vi "Main.vi"() -> ()   [LabVIEW 2017]
doc: "32 channel relay control"
uses:
  Event clusterr.ctl
  EventMsg.ctl
  Sequence cluster.ctl
  SequenceMsg.ctl
  LowLevel cluster.ctl
  LowLevelMsg.ctl
  <vilib>/Utility/file.llb/Read Delimited Spreadsheet (I64).vi
panel:
  out "Current command to Arduino":string
  in  "clear error":bool
  in  "Arduino VISA resource name":refnum<visa-resource-name>
  in  "Exit":bool
  out "ERROR OUT":errorcluster
  in  "Frequency":dbl
  in  "RUN/STOP Signal":bool
  in  "RESET":bool
  out "StopLED":bool
  out "Current step":dbl=-1.0
  in  "Load File":bool
  in  "Path":path
  in  "Next":bool
  in  "Play":bool
  in  "Back":bool
  # "32-channel Relay controller. (C) Michael Shustov. MNFL. 2021"
  # "Sequence control"
  # "Signal generator control"
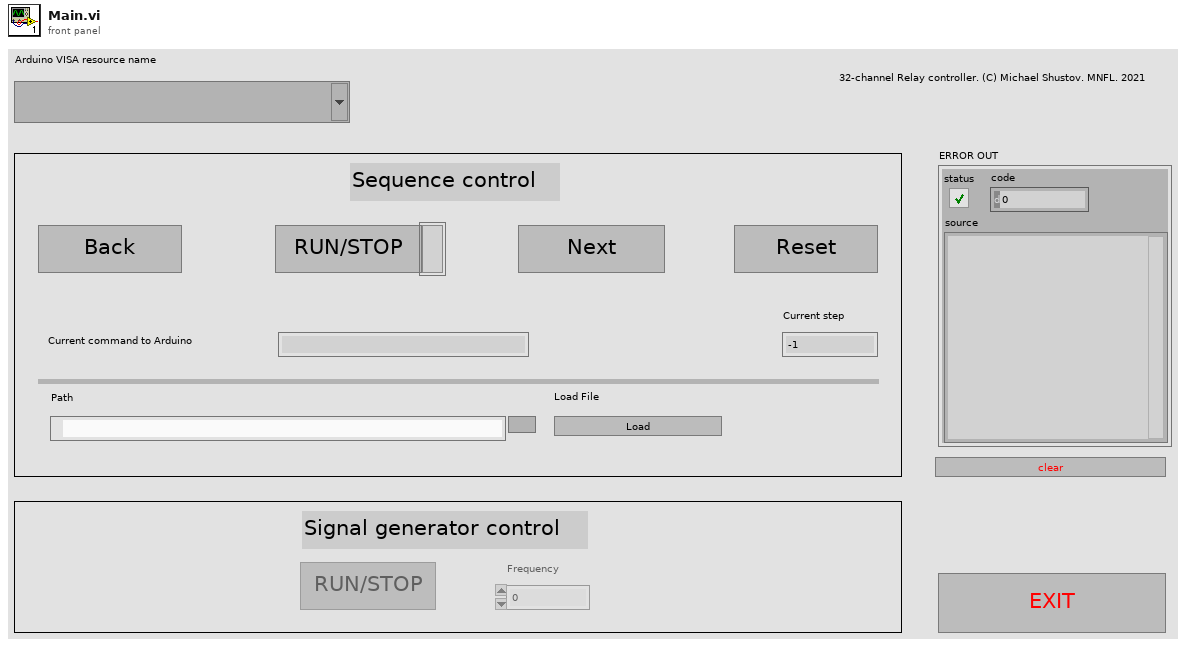
[diagram p1: front panel]
types:
  T1 = cluster{"EventQue":refnum<queue>, "SequenceQue":refnum<queue>, "LowLevelQue":refnum<queue>}
  T2 = cluster{"Back":refnum<vi>, "Play":refnum<vi>, "Next":refnum<vi>, "Load File":refnum<vi>, "RESET":refnum<vi>, "RUN/STOP Signal":refnum<vi>, "Path":refnum<vi>, "StopLED":refnum<vi>, "Current step":refnum<vi>, "Frequency":refnum<vi>, "ERROR OUT":refnum<vi>, "Exit":refnum<vi>, "Arduino VISA resource name":refnum<vi>}
  T3 = typedef "Event clusterr.ctl" = cluster{"EventMsg":T4, "Event string":string}
  T4 = typedef "EventMsg.ctl" = enum16{"Init", "Halt", "Listen"}
  T5 = typedef "Sequence cluster.ctl" = cluster{"SequenceMsg":T6, "Sequence String":string}
  T6 = typedef "SequenceMsg.ctl" = enum16{"Init", "Halt", "Load", "RunStop", "Back", "NextManual", "NextSequenceStep", "Reset"}
  T7 = typedef "LowLevel cluster.ctl" = cluster{"LowLevelMsg":T8, "LowLevel string":string}
  T8 = typedef "LowLevelMsg.ctl" = enum16{"ResetArduinoState", "Init", "Halt", "SetArduinoState", "RunStopSigGen", "Error"}
  T9 = enum8{"Enabled", "Disabled", "Disabled and Grayed Out"}
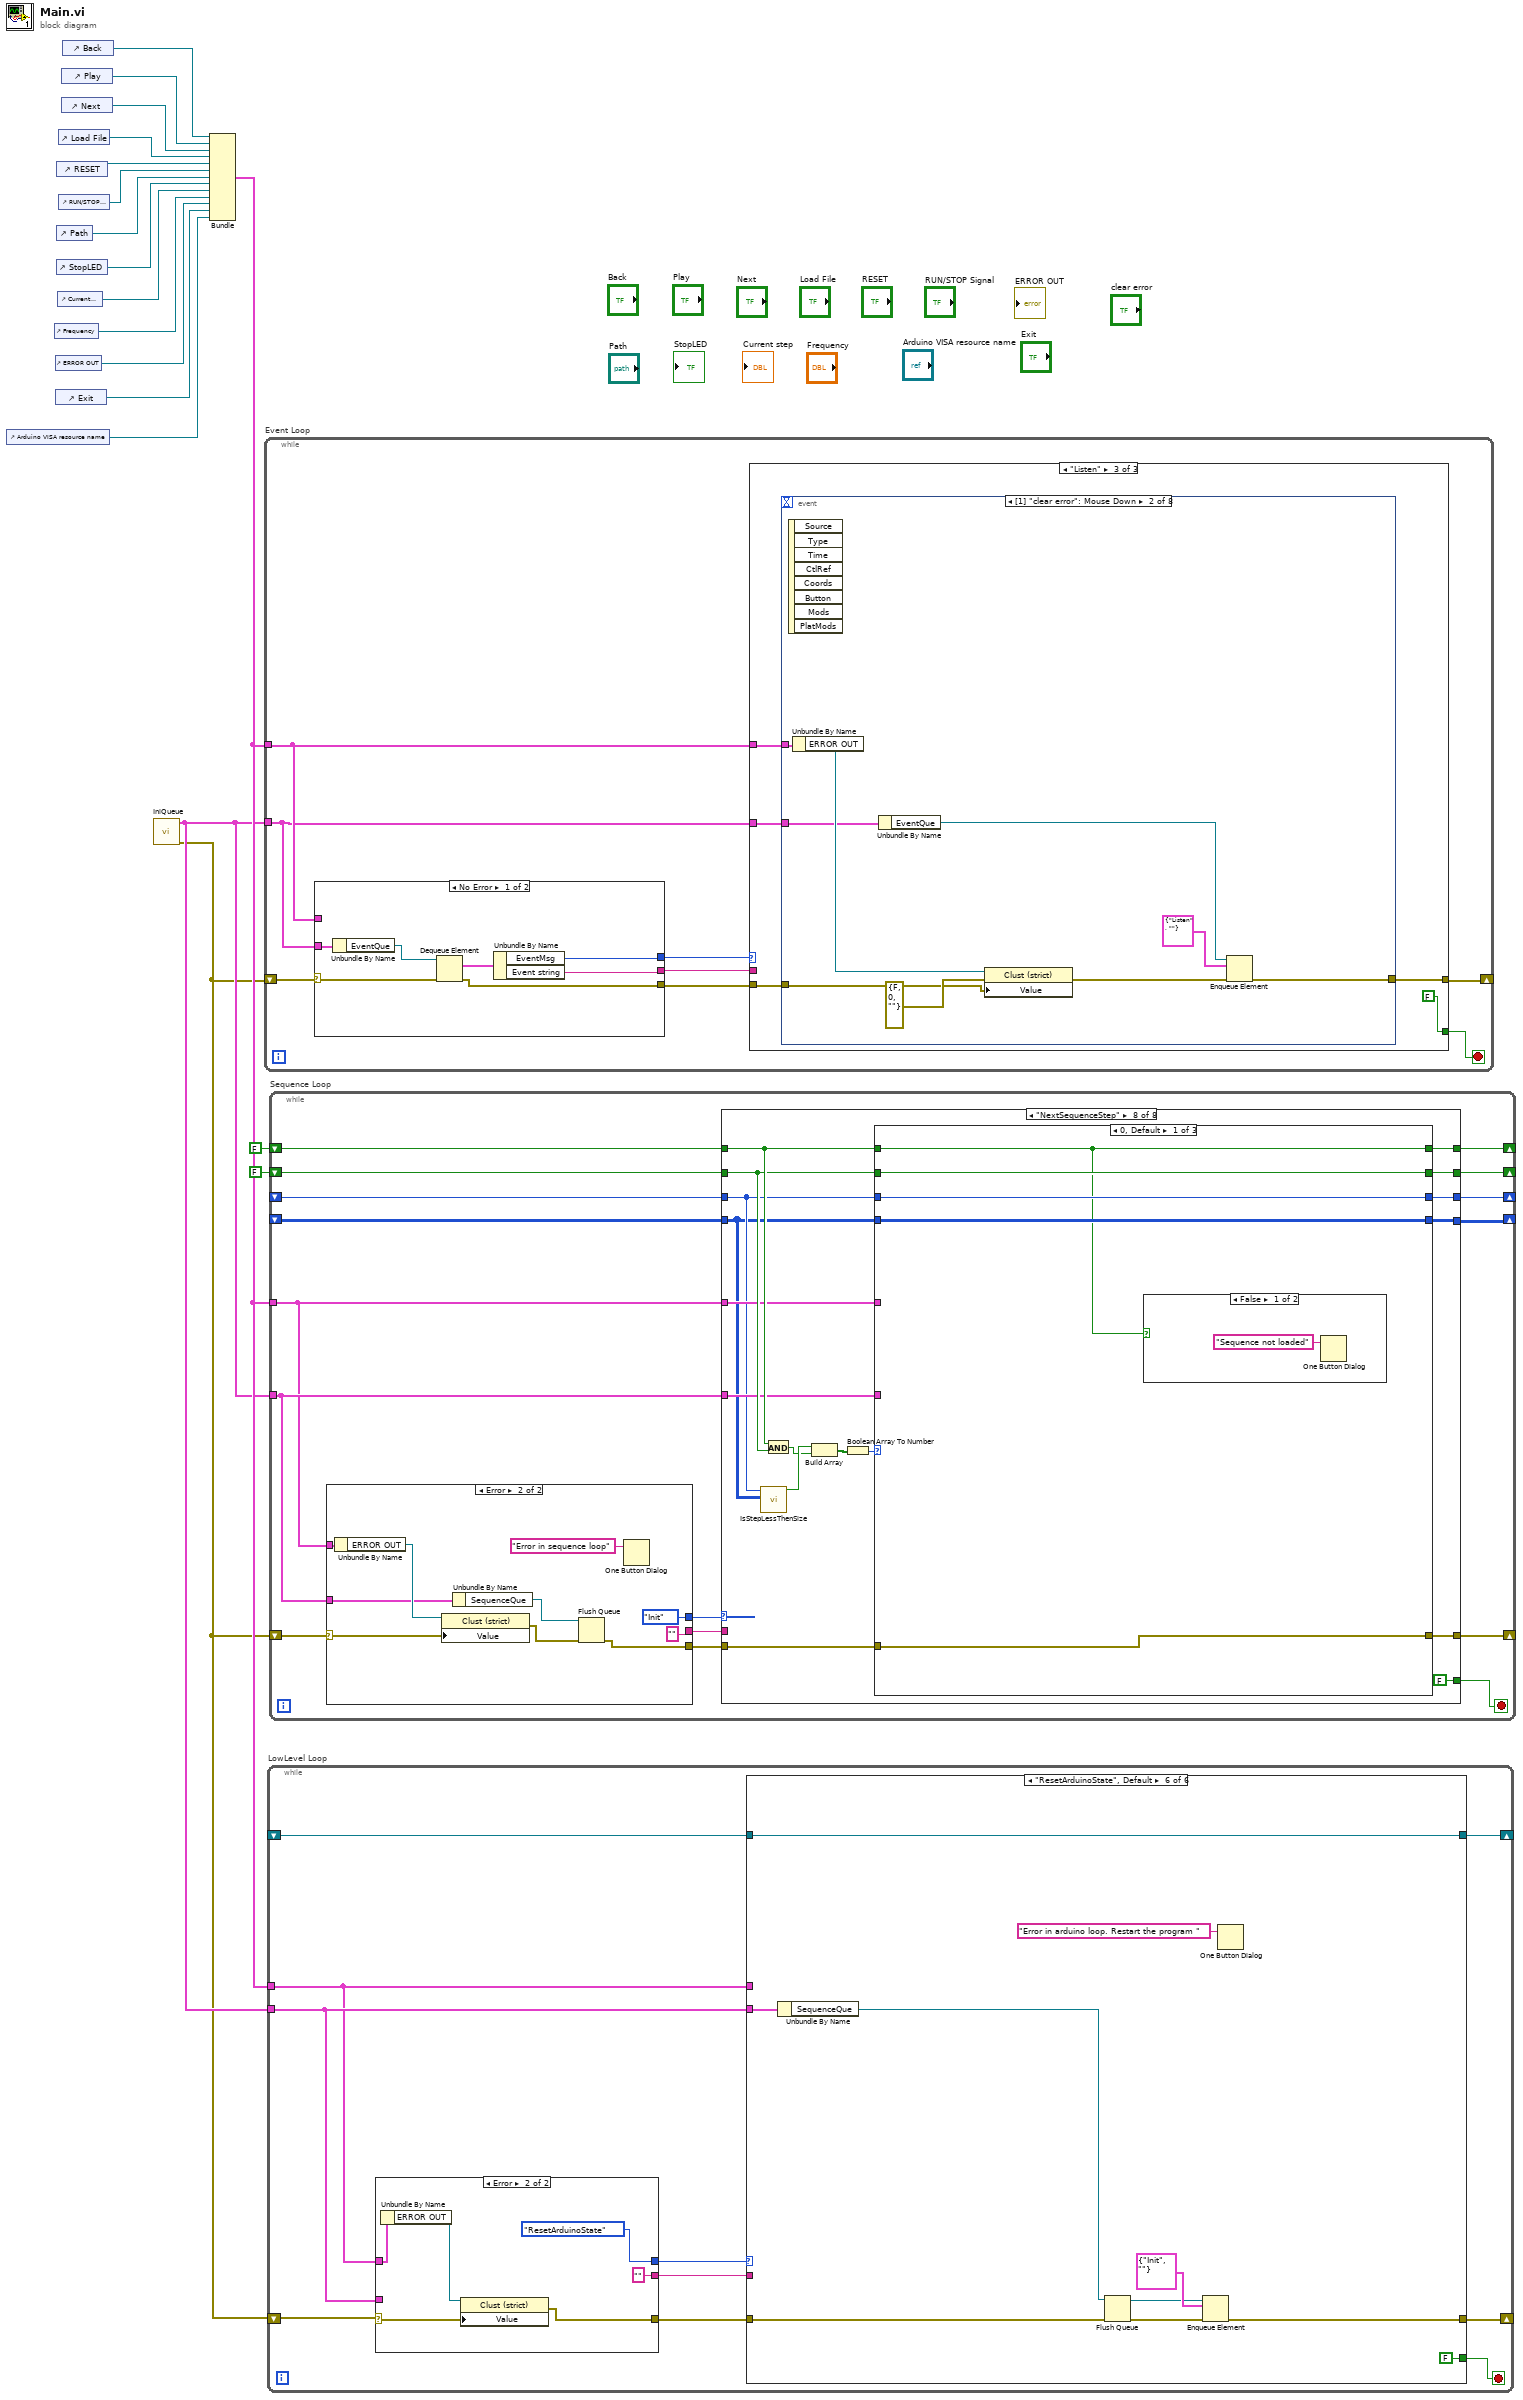
[diagram p0: block diagram]
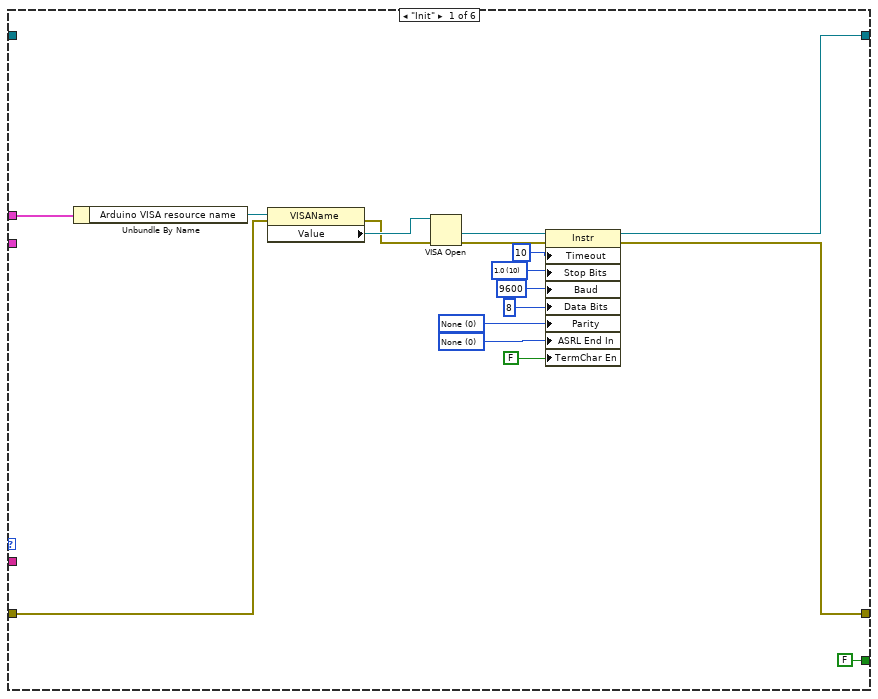
[diagram p2: hidden frame]
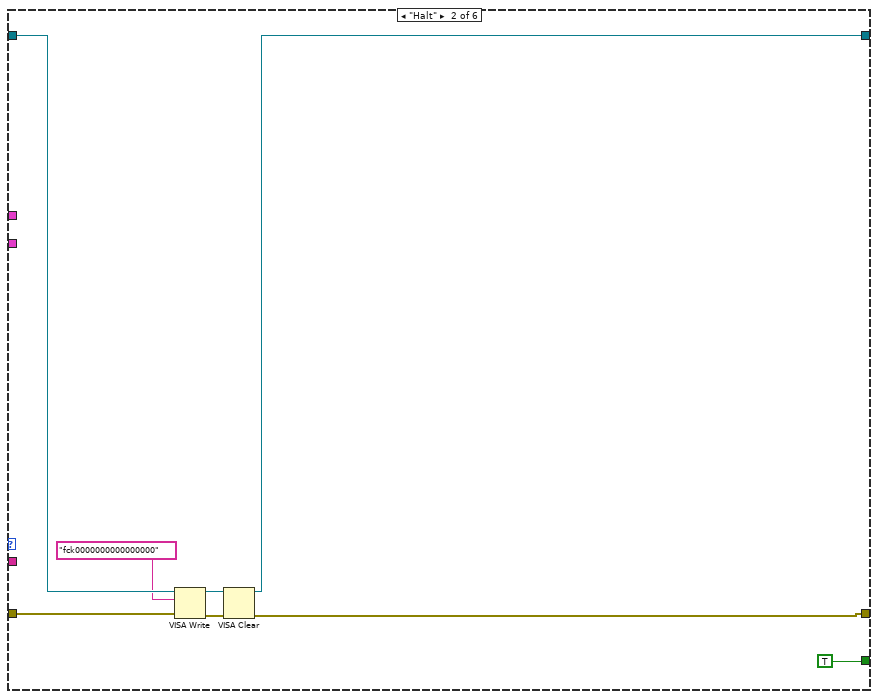
[diagram p3: hidden frame]
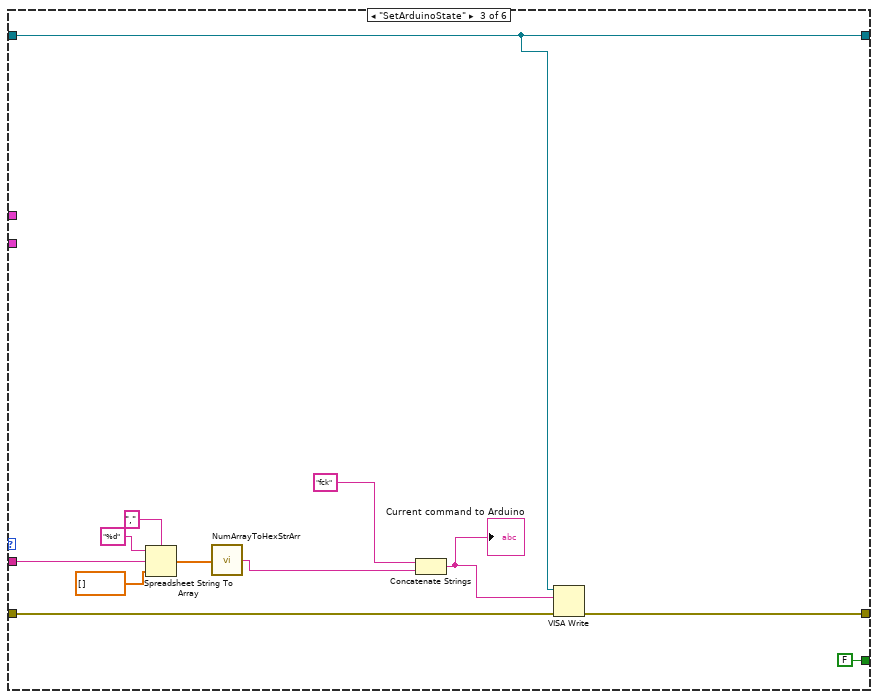
[diagram p4: hidden frame]
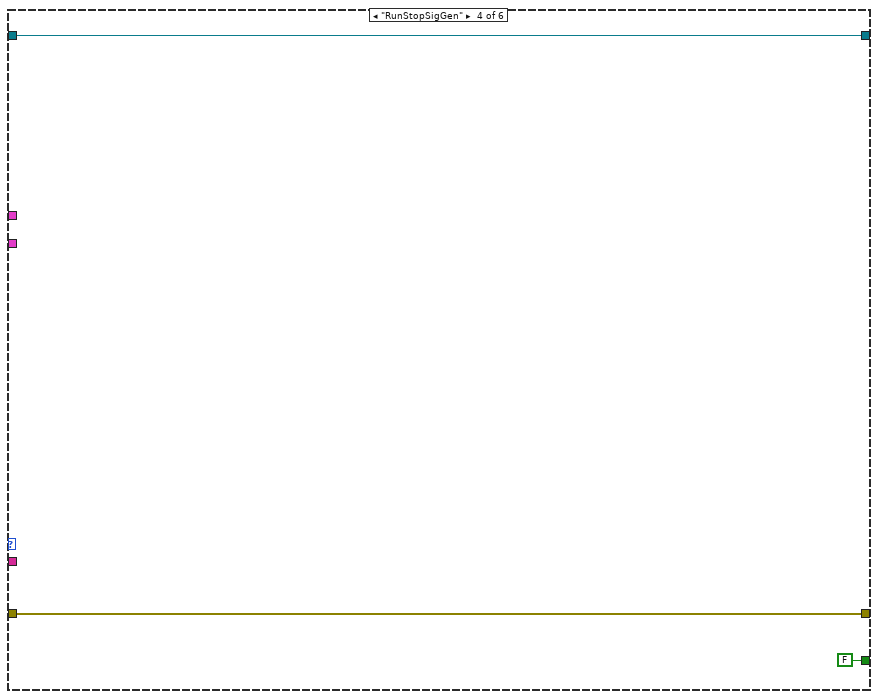
[diagram p5: hidden frame]
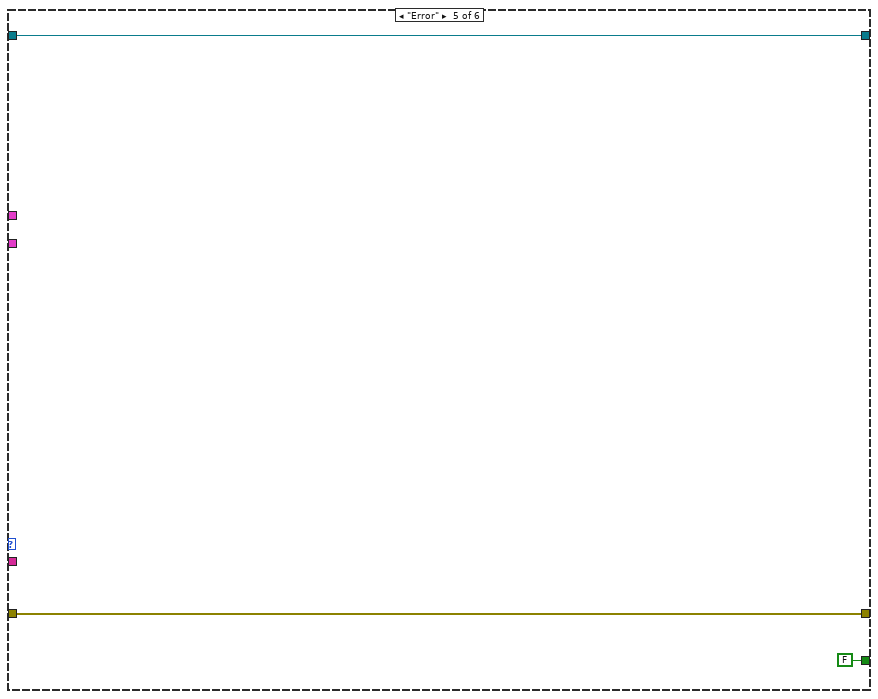
[diagram p6: hidden frame]
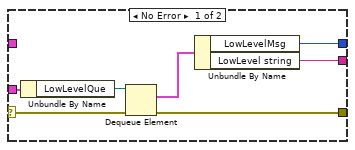
[diagram p7: hidden frame]
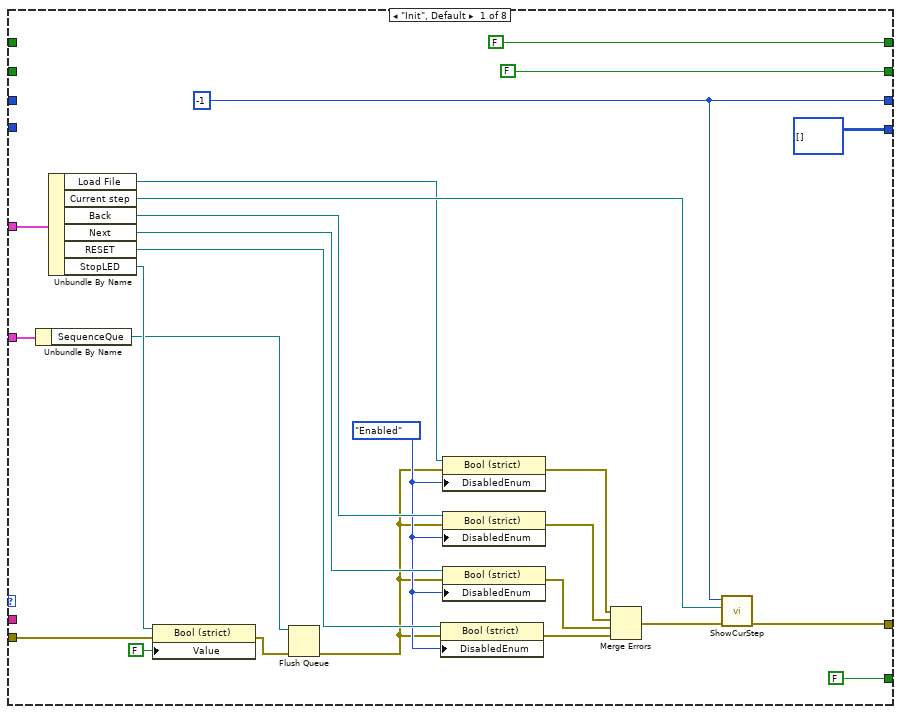
[diagram p8: hidden frame]
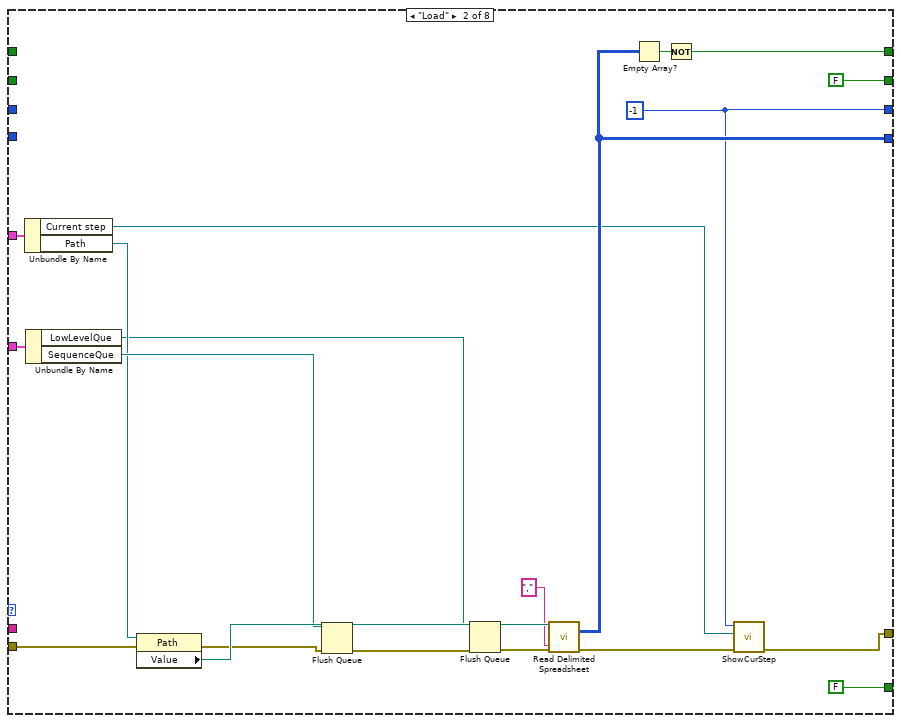
[diagram p9: hidden frame]
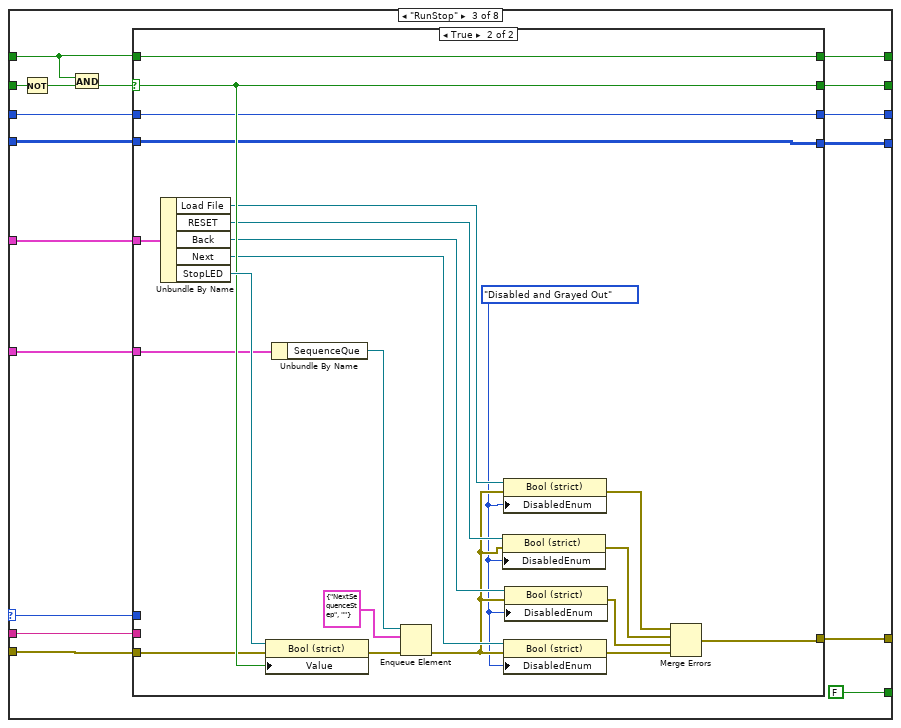
[diagram p10: hidden frame]
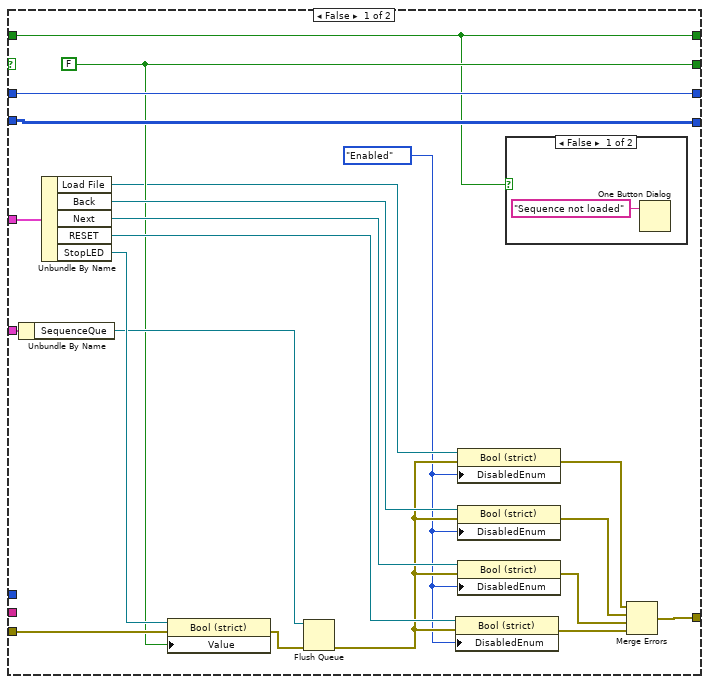
[diagram p11: hidden frame]
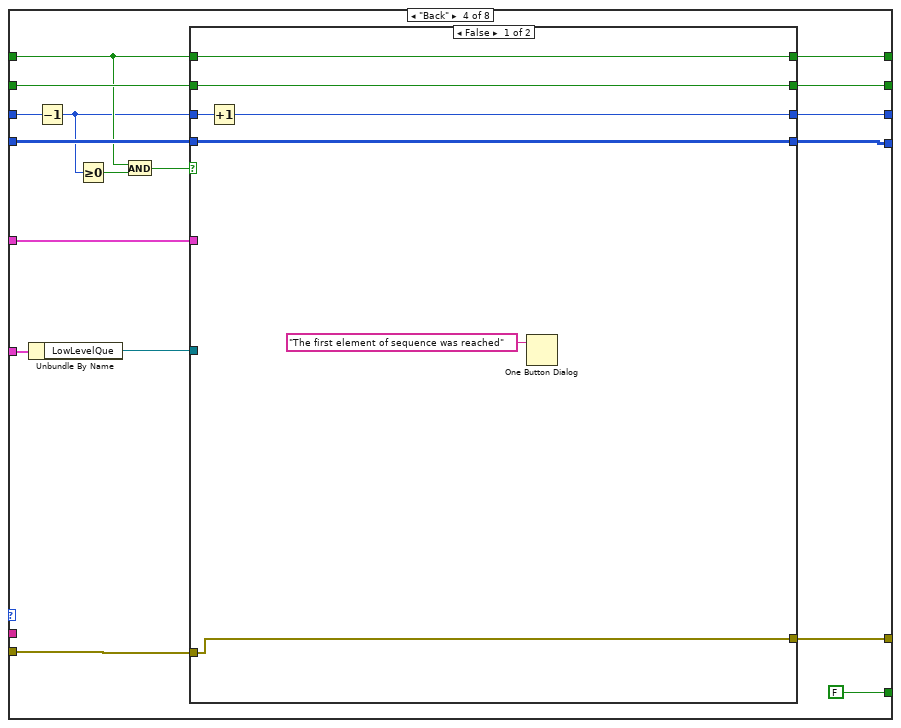
[diagram p13: hidden frame]
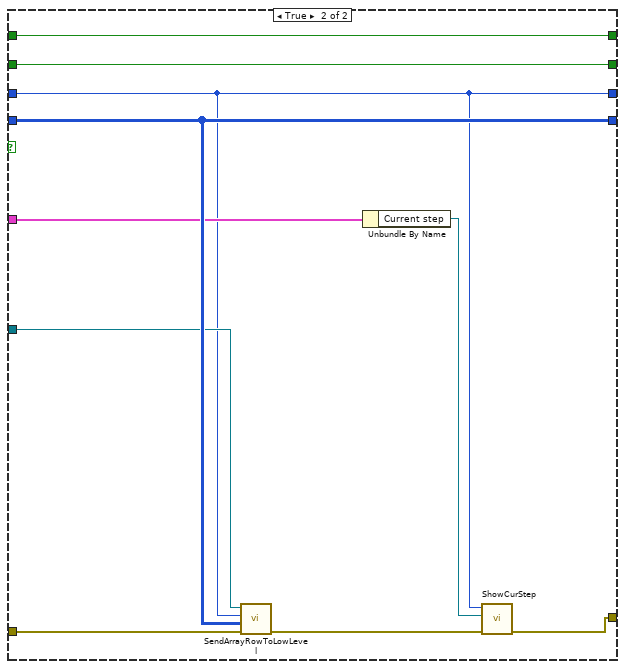
[diagram p14: hidden frame]
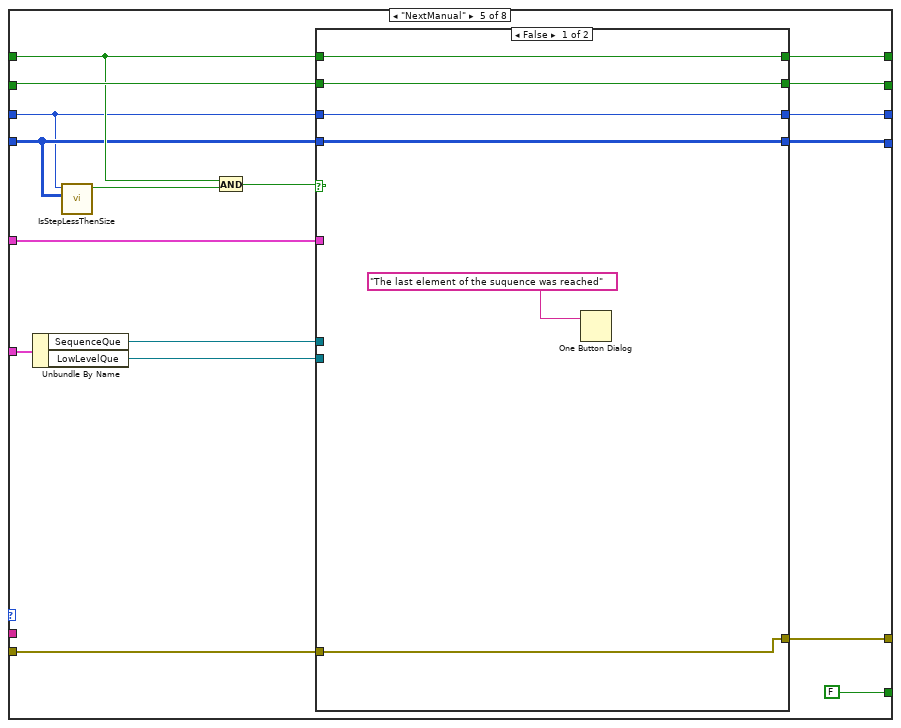
[diagram p15: hidden frame]
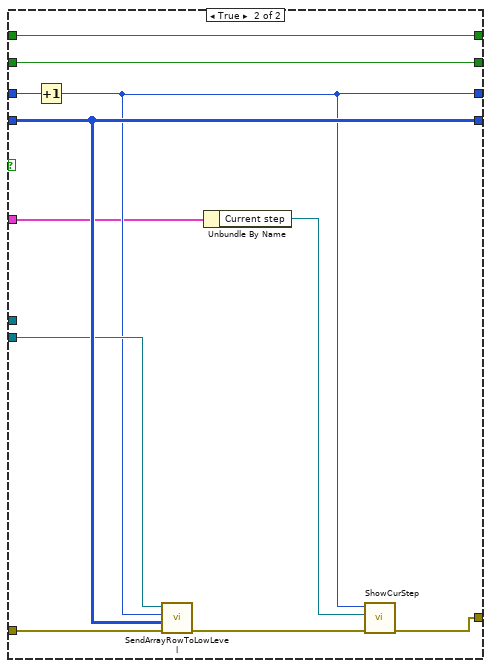
[diagram p16: hidden frame]
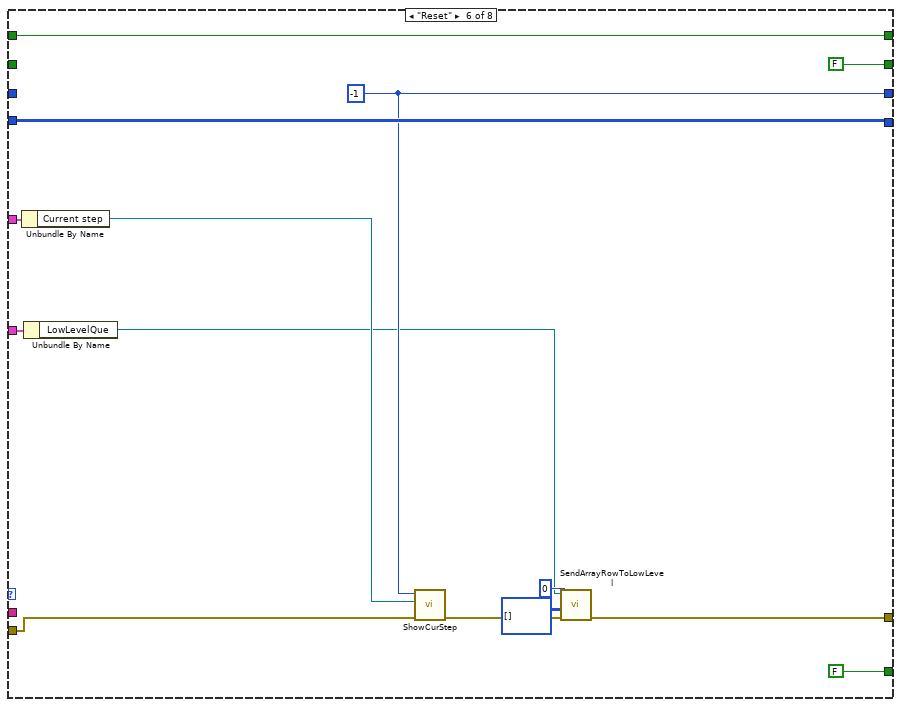
[diagram p17: hidden frame]
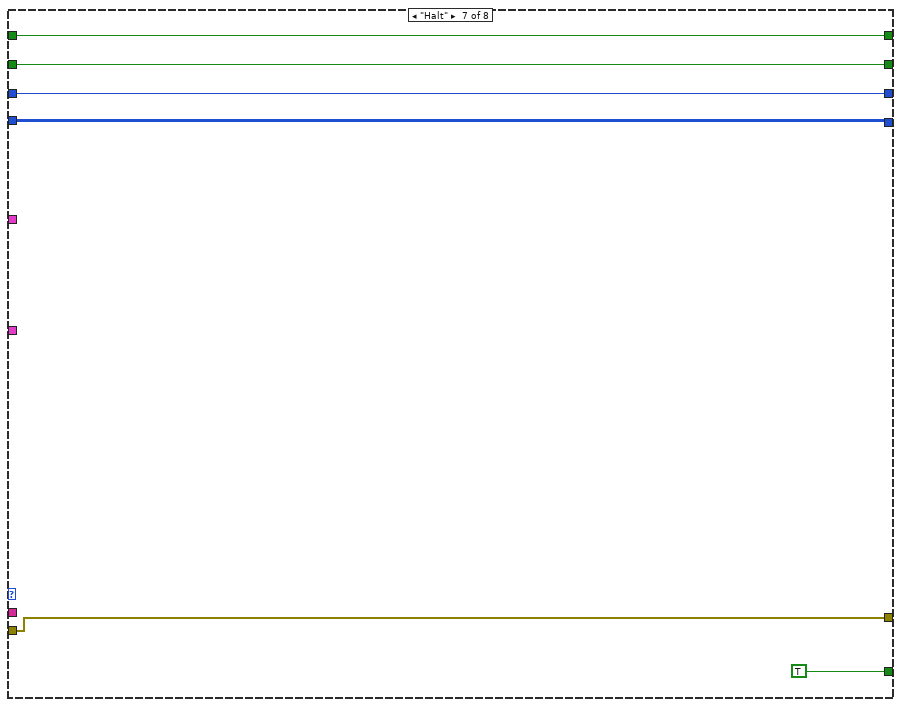
[diagram p18: hidden frame]
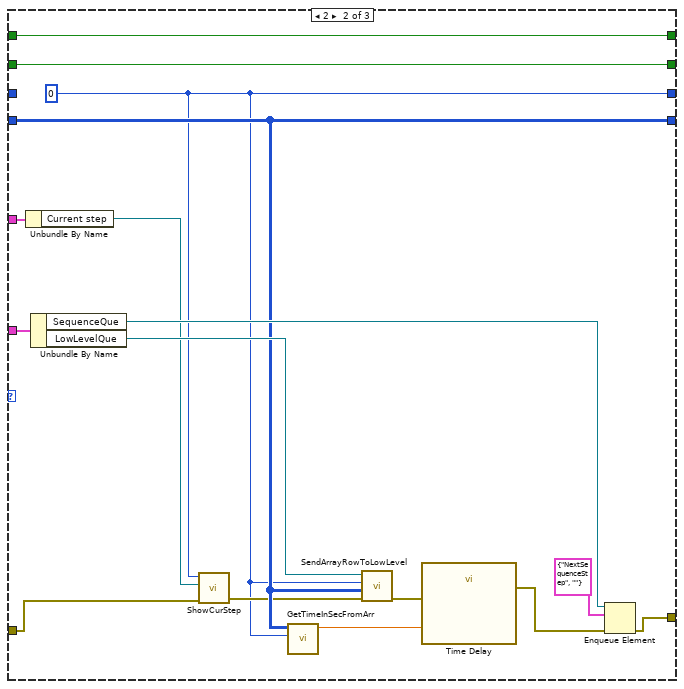
[diagram p20: hidden frame]
diagram:
  n1 = control-ref of="Arduino VISA resource name"() -> (w3:refnum<vi>)
  n2 = control-ref of="Frequency"() -> (w9:refnum<vi>)
  n3 = control-ref of="ERROR OUT"() -> (w7:refnum<vi>)
  n4 = control-ref of="Exit"() -> (w6:refnum<vi>)
  n5 = control-ref of="Path"() -> (w12:refnum<vi>)
  n6 = control-ref of="StopLED"() -> (w11:refnum<vi>)
  n7 = control-ref of="RESET"() -> (w14:refnum<vi>)
  n8 = control-ref of="Current step"() -> (w10:refnum<vi>)
  n9 = control-ref of="Load File"() -> (w15:refnum<vi>)
  n10 = control-ref of="RUN/STOP Signal"() -> (w13:refnum<vi>)
  n11 = control-ref of="Next"() -> (w16:refnum<vi>)
  n12 = control-ref of="Play"() -> (w17:refnum<vi>)
  n13 = control-ref of="Back"() -> (w18:refnum<vi>)
  n14 = call "IniQueue.vi"() -> ("error out"=w4:errorcluster, "Cluster"=w5:T1)  [unwired: 10 in]
  n15 = Bundle("Back"=w18, "Play"=w17, "Next"=w16, "Load File"=w15, "RESET"=w14, "RUN/STOP Signal"=w13, "Path"=w12, "StopLED"=w11, "Current step"=w10, "Frequency"=w9, "ERROR OUT"=w7, "Exit"=w6, "Arduino VISA resource name"=w3) -> (w8:T2)  [unwired: 1 in]
  n16 = while "Event Loop" {
    tunnel: w8 -> [w20]
    tunnel: w5 -> [w19]
    shift-right: [w22] -> _
    shift-left: w4 -> [w21]
    stop <- w23 stop-if-true
    n17 = case shown="No Error" w21 {
      selector: w21 -> [w120 w128]
      tunnel: [w118 w126] -> w26
      tunnel: [w117 w125] -> w25
      tunnel: [w116 w124] -> w24
      tunnel: w20 -> [_ w130]
      tunnel: w19 -> [w115 w122]
      frame No Error {
        n18 = Unbundle By Name(w115) -> ("EventQue"=w114:refnum<queue>)
        n19 = Dequeue Element(queue=w114, error in (no error)=w120) -> (element=w119:T3, error out=w116:errorcluster)  [unwired: 1 in, 2 out]
        n20 = Unbundle By Name(w119) -> ("EventMsg"=w118:T4, "Event string"=w117:string)
      }
      frame Error {
        n21 = Unbundle By Name(w130) -> ("ERROR OUT"=w129:refnum<vi>)
        n22 = Unbundle By Name(w122) -> ("EventQue"=w121:refnum<queue>)
        n23 = Dequeue Element(queue=w121) -> (element=w127:T3, error out=w123:errorcluster)  [unwired: 2 in, 2 out]
        n24 = property class="Clust (strict)"(reference=w129, error in=w123, "Value"=w128) -> (error out=w124:errorcluster)  [unwired: 1 out]
        n25 = Unbundle By Name(w127) -> ("EventMsg"=w126:T4, "Event string"=w125:string)
      }
    }
    n26 = case shown="\"Listen\"" w26 {
      tunnel: w25 -> [_ _ _]
      tunnel: w24 -> [w31 w33 w37]
      tunnel: [FALSE TRUE FALSE] -> w23
      tunnel: [w29 w33 w36] -> w22
      tunnel: w20 -> [_ _ w38]
      tunnel: w19 -> [w28 _ w35]
      frame "Init", Default {
        n27 = Unbundle By Name(w28) -> ("EventQue"=w27:refnum<queue>)
        n28 = Enqueue Element(queue=w27, element=T3 {"EventMsg"=enum."Listen", "Event string"=""}, error in (no error)=w31) -> (error out=w29:errorcluster)  [unwired: 1 in, 2 out]
      }
      frame "Halt" {
      }
      frame "Listen" {
        n29 = event shown="[1] \"clear error\": Mouse Down" {
          selector: _ -> [_ _ _ _ _ _ _ _]
          dyn-events: _ -> [_ _ _ _ _ _ _ _]
          timeout: _ -> [_ _ _ _ _ _ _ _]
          tunnel: w38 -> [_ w56 _ _ _ _ _ _]
          tunnel: w37 -> [w47 w53 w70 w81 w89 w97 w105 w113]
          tunnel: [w43 w50 w61 w77 w86 w93 w101 w110] -> w36
          tunnel: w35 -> [w42 w52 w60 w76 w85 w92 w100 w108]
          event "Back": Mouse Down {
            n30 = event-data() -> ()  [unwired: 1 in, 8 out]
            n31 = Unbundle By Name(w42) -> ("EventQue"=w41:refnum<queue>, "SequenceQue"=w40:refnum<queue>)
            n32 = Enqueue Element(queue=w40, element=T5 {"SequenceMsg"=enum."Back", "Sequence String"=""}, error in (no error)=w47) -> (error out=w44:errorcluster)  [unwired: 1 in, 2 out]
            n33 = Enqueue Element(queue=w41, element=T3 {"EventMsg"=enum."Listen", "Event string"=""}, error in (no error)=w44) -> (error out=w43:errorcluster)  [unwired: 1 in, 2 out]
          }
          event "clear error": Mouse Down {
            n34 = event-data() -> ()  [unwired: 1 in, 8 out]
            n35 = Unbundle By Name(w56) -> ("ERROR OUT"=w55:refnum<vi>)
            n36 = Unbundle By Name(w52) -> ("EventQue"=w49:refnum<queue>)
            n37 = property class="Clust (strict)"(reference=w55, error in=errorcluster {"status"=FALSE, "code"=0, "source"=""} ("error in (no error)"), "Value"=w53) -> (error out=w51:errorcluster)  [unwired: 1 out]
            n38 = Enqueue Element(queue=w49, element=T3 {"EventMsg"=enum."Listen", "Event string"=""}, error in (no error)=w51) -> (error out=w50:errorcluster)  [unwired: 1 in, 2 out]
          }
          event "Exit": Mouse Down {
            n39 = event-data() -> ()  [unwired: 1 in, 8 out]
            n40 = Unbundle By Name(w60) -> ("EventQue"=w59:refnum<queue>, "SequenceQue"=w58:refnum<queue>, "LowLevelQue"=w57:refnum<queue>)
            n41 = Flush Queue(queue=w59, error in (no error)=w70) -> (queue out=w73:refnum<queue>, error out=w71:errorcluster)  [unwired: 1 out]
            n42 = Enqueue Element(queue=w73, element=T3 {"EventMsg"=enum."Halt", "Event string"=""}, error in (no error)=w71) -> (error out=w69:errorcluster)  [unwired: 1 in, 2 out]
            n43 = Flush Queue(queue=w58, error in (no error)=w69) -> (queue out=w68:refnum<queue>, error out=w67:errorcluster)  [unwired: 1 out]
            n44 = Enqueue Element(queue=w68, element=T5 {"SequenceMsg"=enum."Halt", "Sequence String"=""}, error in (no error)=w67) -> (error out=w65:errorcluster)  [unwired: 1 in, 2 out]
            n45 = Flush Queue(queue=w57, error in (no error)=w65) -> (queue out=w64:refnum<queue>, error out=w63:errorcluster)  [unwired: 1 out]
            n46 = Enqueue Element(queue=w64, element=T7 {"LowLevelMsg"=enum."Halt", "LowLevel string"=""}, error in (no error)=w63) -> (error out=w61:errorcluster)  [unwired: 1 in, 2 out]
          }
          event "Play": Mouse Down {
            n47 = event-data() -> ()  [unwired: 1 in, 8 out]
            n48 = Unbundle By Name(w76) -> ("EventQue"=w74:refnum<queue>, "SequenceQue"=w75:refnum<queue>)
            n49 = Enqueue Element(queue=w75, element=T5 {"SequenceMsg"=enum."RunStop", "Sequence String"=""}, error in (no error)=w81) -> (error out=w78:errorcluster)  [unwired: 1 in, 2 out]
            n50 = Enqueue Element(queue=w74, element=T3 {"EventMsg"=enum."Listen", "Event string"=""}, error in (no error)=w78) -> (error out=w77:errorcluster)  [unwired: 1 in, 2 out]
          }
          event "Next": Mouse Down {
            n51 = event-data() -> ()  [unwired: 1 in, 8 out]
            n52 = Unbundle By Name(w85) -> ("EventQue"=w84:refnum<queue>, "SequenceQue"=w83:refnum<queue>)
            n53 = Enqueue Element(queue=w83, element=T5 {"SequenceMsg"=enum."NextManual", "Sequence String"=""}, error in (no error)=w89) -> (error out=w87:errorcluster)  [unwired: 1 in, 2 out]
            n54 = Enqueue Element(queue=w84, element=T3 {"EventMsg"=enum."Listen", "Event string"=""}, error in (no error)=w87) -> (error out=w86:errorcluster)  [unwired: 1 in, 2 out]
          }
          event "Load File": Mouse Down {
            n55 = event-data() -> ()  [unwired: 1 in, 8 out]
            n56 = Unbundle By Name(w92) -> ("EventQue"=w90:refnum<queue>, "SequenceQue"=w91:refnum<queue>)
            n57 = Enqueue Element(queue=w91, element=T5 {"SequenceMsg"=enum."Load", "Sequence String"=""}, error in (no error)=w97) -> (error out=w94:errorcluster)  [unwired: 1 in, 2 out]
            n58 = Enqueue Element(queue=w90, element=T3 {"EventMsg"=enum."Listen", "Event string"=""}, error in (no error)=w94) -> (error out=w93:errorcluster)  [unwired: 1 in, 2 out]
          }
          event "RESET": Mouse Down {
            n59 = event-data() -> ()  [unwired: 1 in, 8 out]
            n60 = Unbundle By Name(w100) -> ("EventQue"=w99:refnum<queue>, "SequenceQue"=w98:refnum<queue>)
            n61 = Enqueue Element(queue=w98, element=T5 {"SequenceMsg"=enum."Reset", "Sequence String"=""}, error in (no error)=w105) -> (error out=w102:errorcluster)  [unwired: 1 in, 2 out]
            n62 = Enqueue Element(queue=w99, element=T3 {"EventMsg"=enum."Listen", "Event string"=""}, error in (no error)=w102) -> (error out=w101:errorcluster)  [unwired: 1 in, 2 out]
          }
          event "RUN/STOP Signal": Mouse Down {
            n63 = event-data() -> ()  [unwired: 1 in, 8 out]
            n64 = Unbundle By Name(w108) -> ("EventQue"=w106:refnum<queue>, "LowLevelQue"=w107:refnum<queue>)
            n65 = Enqueue Element(queue=w107, element=T7 {"LowLevelMsg"=enum."RunStopSigGen", "LowLevel string"=""}, error in (no error)=w113) -> (error out=w111:errorcluster)  [unwired: 1 in, 2 out]
            n66 = Enqueue Element(queue=w106, element=T3 {"EventMsg"=enum."Listen", "Event string"=""}, error in (no error)=w111) -> (error out=w110:errorcluster)  [unwired: 1 in, 2 out]
          }
        }
      }
    }
  }
  n67 = while "LowLevel Loop" {
    tunnel: w8 -> [w134]
    tunnel: w5 -> [w135]
    shift-right: [w131] -> _
    shift-left: w4 -> [w136]
    shift-right: [w133] -> _
    shift-left: _ -> [w132]
    stop <- w137 stop-if-true
    n68 = case shown="Error" w136 {
      selector: w136 -> [w199 w204]
      tunnel: w135 -> [w200 _]
      tunnel: [w197 LowLevelMsg."ResetArduinoState" ("LowLevelMsg")] -> w138
      tunnel: [w196 "" ("LowLevel string")] -> w140
      tunnel: [w195 w203] -> w139
      tunnel: w134 -> [_ w206]
      frame No Error {
        n69 = Unbundle By Name(w200) -> ("LowLevelQue"=w194:refnum<queue>)
        n70 = Dequeue Element(queue=w194, error in (no error)=w199) -> (element=w198:T7, error out=w195:errorcluster)  [unwired: 1 in, 2 out]
        n71 = Unbundle By Name(w198) -> ("LowLevelMsg"=w197:T8, "LowLevel string"=w196:string)
      }
      frame Error {
        n72 = Unbundle By Name(w206) -> ("ERROR OUT"=w205:refnum<vi>)
        n73 = property class="Clust (strict)"(reference=w205, "Value"=w204) -> (error out=w203:errorcluster)  [unwired: 1 in, 1 out]
      }
    }
    n74 = case shown="\"ResetArduinoState\", Default" w138 {
      tunnel: w140 -> [_ _ w177 _ _ _]
      tunnel: w139 -> [w155 w159 w169 w179 w182 w187]
      tunnel: [FALSE TRUE FALSE FALSE FALSE FALSE] -> w137
      tunnel: [w142 w164 w166 w179 w182 w190] -> w131
      tunnel: w135 -> [_ _ _ _ _ w191]
      tunnel: w134 -> [w157 _ _ _ _ _]
      tunnel: [w141 w163 w167 w180 w183 w193] -> w133
      tunnel: w132 -> [_ w160 w167 w180 w183 w193]
      frame "Init" {
        w147 = u16 10 items=["1.0"=10, "1.5"=15, "2.0"=20] ("Serial Settings:Stop Bits")
        w150 = u16 0 items=["None", "Odd", "Even", "Mark", "Space"] ("Serial Settings:Parity")
        w151 = u16 0 items=["None", "Last Bit", "TermChar"] ("Serial Settings:End Mode for Reads")
        n75 = Unbundle By Name(w157) -> ("Arduino VISA resource name"=w156:refnum<vi>)
        n76 = property class="VISAName"(reference=w156, error in=w155) -> (error out=w145:errorcluster, "Value"=w146:refnum<visa-resource-name>)  [unwired: 1 out]
        n77 = VISA Open(error in (no error)=w145, VISA resource name=w146) -> (VISA resource name=w143:refnum<visa-resource-name>, error out=w144:errorcluster)  [unwired: 3 in]
        n78 = property class="Instr"(reference=w143, error in=w144, "Timeout"=u32 10 ("General Settings:Timeout Value"), "Stop Bits"=w147, "Baud"=u32 9600 ("Serial Settings:Baud Rate"), "Data Bits"=u16 8 ("Serial Settings:Data Bits"), "Parity"=w150, "ASRL End In"=w151, "TermChar En"=FALSE ("Message Based Settings:Termination Character Enable")) -> (reference out=w141:refnum<visa-resource-name>, error out=w142:errorcluster)
      }
      frame "Halt" {
        n79 = VISA Write(VISA resource name=w160, write buffer="fck0000000000000000", error in (no error)=w159) -> (VISA resource name out=w161:refnum<visa-resource-name>, error out=w162:errorcluster)  [unwired: 1 out]
        n80 = VISA Clear(VISA resource name=w161, error in (no error)=w162) -> (VISA resource name out=w163:refnum<visa-resource-name>, error out=w164:errorcluster)
      }
      frame "SetArduinoState" {
        n81 = Spreadsheet String To Array(delimiter (Tab)=",", format string="%d", spreadsheet string=w177, array type (2D Dbl)=dbl[] []) -> (array=w173:dbl[])
        n82 = call "NumArrayToHexStrArr.vi"("Array of numbers"=w173) -> ("concatenated string"=w170:string)
        n83 = Concatenate Strings("fck" ("string"), w170) -> (w168:string)
        "Current command to Arduino" <- w168
        n84 = VISA Write(VISA resource name=w167, write buffer=w168, error in (no error)=w169) -> (error out=w166:errorcluster)  [unwired: 2 out]
      }
      frame "RunStopSigGen" {
      }
      frame "Error" {
      }
      frame "ResetArduinoState", Default {
        n85 = Unbundle By Name(w191) -> ("SequenceQue"=w186:refnum<queue>)
        n86 = Flush Queue(queue=w186, error in (no error)=w187) -> (queue out=w185:refnum<queue>, error out=w188:errorcluster)  [unwired: 1 out]
        n87 = Enqueue Element(queue=w185, element=T5 {"SequenceMsg"=enum."Init", "Sequence String"=""}, error in (no error)=w188) -> (error out=w190:errorcluster)  [unwired: 1 in, 2 out]
        n88 = One Button Dialog(message="Error in arduino loop. Restart the program ") -> ()  [unwired: 1 in, 1 out]
      }
    }
  }
  n89 = while "Sequence Loop" {
    tunnel: w8 -> [w209]
    tunnel: w5 -> [w212]
    shift-right: [w213] -> _
    shift-left: w4 -> [w222]
    shift-right: [w218] -> _
    shift-left: FALSE -> [w217]
    shift-right: [w216] -> _
    shift-left: _ -> [w207]
    shift-right: [w214] -> _
    shift-left: _ -> [w208]
    shift-right: [w211] -> _
    shift-left: FALSE -> [w210]
    stop <- w219 stop-if-true
    n90 = case shown="Error" w222 {
      selector: w222 -> [w477 w487]
      tunnel: w212 -> [w479 w486]
      tunnel: w209 -> [_ w489]
      tunnel: [w475 SequenceMsg."Init" ("SequenceMsg")] -> w220
      tunnel: [w474 "" ("Sequence String")] -> w221
      tunnel: [w473 w483] -> w215
      frame No Error {
        n91 = Unbundle By Name(w479) -> ("SequenceQue"=w478:refnum<queue>)
        n92 = Dequeue Element(queue=w478, error in (no error)=w477) -> (element=w476:T5, error out=w473:errorcluster)  [unwired: 1 in, 2 out]
        n93 = Unbundle By Name(w476) -> ("SequenceMsg"=w475:T6, "Sequence String"=w474:string)
      }
      frame Error {
        n94 = Unbundle By Name(w489) -> ("ERROR OUT"=w488:refnum<vi>)
        n95 = property class="Clust (strict)"(reference=w488, "Value"=w487) -> (error out=w485:errorcluster)  [unwired: 1 in, 1 out]
        n96 = Unbundle By Name(w486) -> ("SequenceQue"=w484:refnum<queue>)
        n97 = Flush Queue(queue=w484, error in (no error)=w485) -> (error out=w483:errorcluster)  [unwired: 2 out]
        n98 = One Button Dialog(message="Error in sequence loop") -> ()  [unwired: 1 in, 1 out]
      }
    }
    n99 = case shown="\"NextSequenceStep\"" w220 {
      selector: w220 -> [_ _ w277 _ _ _ _ _]
      tunnel: w221 -> [_ _ w278 _ _ _ _ _]
      tunnel: [FALSE FALSE FALSE FALSE FALSE FALSE TRUE FALSE] -> w219
      tunnel: [FALSE FALSE w280 w343 w376 FALSE w413 w428] -> w218
      tunnel: w217 -> [_ _ w284 w344 w377 _ w413 w429]
      tunnel: w207 -> [_ _ w283 w340 w364 _ w412 w420]
      tunnel: [w228 w252 w274 w335 w374 w403 w412 w427] -> w216
      tunnel: w215 -> [w232 w267 w279 w332 w373 w405 w415 w424]
      tunnel: [i64[][] [] ("all rows") w260 w273 w342 w375 w409 w411 w426] -> w214
      tunnel: w208 -> [_ _ w282 w341 w365 w409 w411 w419]
      tunnel: [w227 w253 w276 w331 w372 w401 w415 w423] -> w213
      tunnel: w212 -> [w233 w262 w281 w334 w371 w398 _ w425]
      tunnel: [FALSE w258 w269 w345 w378 w410 w414 w430] -> w211
      tunnel: w210 -> [_ _ w270 w339 w368 w410 w414 w431]
      tunnel: w209 -> [w234 w257 w268 w329 w366 w406 _ w421]
      frame "Init", Default {
        w228 = -1
        w226 = T9."Enabled" ("Disabled")
        n100 = Unbundle By Name(w233) -> ("SequenceQue"=w242:refnum<queue>)
        n101 = Unbundle By Name(w234) -> ("Load File"=w224:refnum<vi>, "Current step"=w229:refnum<vi>, "Back"=w240:refnum<vi>, "Next"=w239:refnum<vi>, "RESET"=w238:refnum<vi>, "StopLED"=w243:refnum<vi>)
        n102 = property class="Bool (strict)"(reference=w243, error in=w232, "Value"=FALSE) -> (error out=w241:errorcluster)  [unwired: 1 out]
        n103 = Flush Queue(queue=w242, error in (no error)=w241) -> (error out=w225:errorcluster)  [unwired: 2 out]
        n104 = property class="Bool (strict)"(reference=w238, error in=w225, "DisabledEnum"=w226) -> (error out=w235:errorcluster)  [unwired: 1 out]
        n105 = property class="Bool (strict)"(reference=w224, error in=w225, "DisabledEnum"=w226) -> (error out=w223:errorcluster)  [unwired: 1 out]
        n106 = property class="Bool (strict)"(reference=w240, error in=w225, "DisabledEnum"=w226) -> (error out=w237:errorcluster)  [unwired: 1 out]
        n107 = property class="Bool (strict)"(reference=w239, error in=w225, "DisabledEnum"=w226) -> (error out=w236:errorcluster)  [unwired: 1 out]
        n108 = Merge Errors(w223, w237, w236, w235) -> (w230:errorcluster)
        n109 = call "ShowCurStep.vi"("error in (no error)"=w230, "Step indicator reference"=w229, "Current step"=w228) -> ("error out"=w227:errorcluster)  [unwired: 8 in]
      }
      frame "Load" {
        w252 = -1
        n110 = Unbundle By Name(w257) -> ("Current step"=w251:refnum<vi>, "Path"=w256:refnum<vi>)
        n111 = Unbundle By Name(w262) -> ("LowLevelQue"=w254:refnum<queue>, "SequenceQue"=w261:refnum<queue>)
        n112 = property class="Path"(reference=w256, error in=w267) -> (error out=w250:errorcluster, "Value"=w266:path)  [unwired: 1 out]
        n113 = Flush Queue(queue=w261, error in (no error)=w250) -> (error out=w255:errorcluster)  [unwired: 2 out]
        n114 = Flush Queue(queue=w254, error in (no error)=w255) -> (error out=w248:errorcluster)  [unwired: 2 out]
        n115 = call-poly <vilib>:"Read Delimited Spreadsheet.vi"("file path (dialog if empty)"=w266, "error in (no error)"=w248, "delimiter (\\t)"="," ("delimiter (\\t)")) -> ("all rows"=w260:i64[][], "error out"=w249:errorcluster)  [unwired: 7 in, 4 out]
        n116 = Empty Array?(array=w260) -> (empty?=w259:bool)
        n117 = Not(x=w259) -> (.not. x?=w258:bool)
        n118 = call "ShowCurStep.vi"("error in (no error)"=w249, "Step indicator reference"=w251, "Current step"=w252) -> ("error out"=w253:errorcluster)  [unwired: 8 in]
      }
      frame "RunStop" {
        n119 = Not(x=w284) -> (.not. x?=w272:bool)
        n120 = And(x=w270, y=w272) -> (x .and. y?=w271:bool)
        n121 = case shown="True" w271 {
          selector: w271 -> [_ w327]
          tunnel: w283 -> [w303 w322]
          tunnel: w282 -> [w302 w321]
          tunnel: w281 -> [w301 w325]
          tunnel: [w290 w327] -> w280
          tunnel: w279 -> [w304 w326]
          tunnel: w278 -> [_ _]
          tunnel: w277 -> [_ _]
          tunnel: [w294 w308] -> w276
          tunnel: [w303 w322] -> w274
          tunnel: [w302 w321] -> w273
          tunnel: w270 -> [w289 w317]
          tunnel: [w289 w317] -> w269
          tunnel: w268 -> [w291 w315]
          frame False {
            w290 = FALSE
            w286 = T9."Enabled" ("Disabled")
            n122 = Unbundle By Name(w301) -> ("SequenceQue"=w300:refnum<queue>)
            n123 = Unbundle By Name(w291) -> ("Load File"=w288:refnum<vi>, "Back"=w298:refnum<vi>, "Next"=w297:refnum<vi>, "RESET"=w296:refnum<vi>, "StopLED"=w305:refnum<vi>)
            n124 = property class="Bool (strict)"(reference=w305, error in=w304, "Value"=w290) -> (error out=w299:errorcluster)  [unwired: 1 out]
            n125 = Flush Queue(queue=w300, error in (no error)=w299) -> (error out=w287:errorcluster)  [unwired: 2 out]
            n126 = property class="Bool (strict)"(reference=w296, error in=w287, "DisabledEnum"=w286) -> (error out=w292:errorcluster)  [unwired: 1 out]
            n127 = property class="Bool (strict)"(reference=w288, error in=w287, "DisabledEnum"=w286) -> (error out=w285:errorcluster)  [unwired: 1 out]
            n128 = property class="Bool (strict)"(reference=w298, error in=w287, "DisabledEnum"=w286) -> (error out=w295:errorcluster)  [unwired: 1 out]
            n129 = property class="Bool (strict)"(reference=w297, error in=w287, "DisabledEnum"=w286) -> (error out=w293:errorcluster)  [unwired: 1 out]
            n130 = case shown="False" w289 {
              frame False {
                n131 = One Button Dialog(message="Sequence not loaded") -> ()  [unwired: 1 in, 1 out]
              }
              frame True {
              }
            }
            n132 = Merge Errors(w285, w295, w293, w292) -> (w294:errorcluster)
          }
          frame True {
            w307 = T9."Disabled and Grayed Out" ("Disabled")
            n133 = Unbundle By Name(w315) -> ("Load File"=w314:refnum<vi>, "RESET"=w320:refnum<vi>, "Back"=w319:refnum<vi>, "Next"=w318:refnum<vi>, "StopLED"=w328:refnum<vi>)
            n134 = property class="Bool (strict)"(reference=w328, error in=w326, "Value"=w327) -> (error out=w323:errorcluster)  [unwired: 1 out]
            n135 = Unbundle By Name(w325) -> ("SequenceQue"=w324:refnum<queue>)
            n136 = Enqueue Element(queue=w324, element=T5 {"SequenceMsg"=enum."NextSequenceStep", "Sequence String"=""}, error in (no error)=w323) -> (error out=w313:errorcluster)  [unwired: 1 in, 2 out]
            n137 = property class="Bool (strict)"(reference=w320, error in=w313, "DisabledEnum"=w307) -> (error out=w310:errorcluster)  [unwired: 1 out]
            n138 = property class="Bool (strict)"(reference=w314, error in=w313, "DisabledEnum"=w307) -> (error out=w309:errorcluster)  [unwired: 1 out]
            n139 = property class="Bool (strict)"(reference=w318, error in=w313, "DisabledEnum"=w307) -> (error out=w312:errorcluster)  [unwired: 1 out]
            n140 = property class="Bool (strict)"(reference=w319, error in=w313, "DisabledEnum"=w307) -> (error out=w311:errorcluster)  [unwired: 1 out]
            n141 = Merge Errors(w309, w310, w311, w312) -> (w308:errorcluster)
          }
        }
      }
      frame "Back" {
        n142 = Unbundle By Name(w334) -> ("LowLevelQue"=w333:refnum<queue>)
        n143 = Decrement(x=w340) -> (x-1=w336:i32)
        n144 = Greater Or Equal To 0?(x=w336) -> (x >= 0?=w338:bool)
        n145 = And(x=w339, y=w338) -> (x .and. y?=w337:bool)
        n146 = case shown="False" w337 {
          tunnel: [w348 w361] -> w345
          tunnel: [w349 w362] -> w343
          tunnel: w344 -> [w349 w362]
          tunnel: w341 -> [w350 w360]
          tunnel: [w350 w360] -> w342
          tunnel: w339 -> [w348 w361]
          tunnel: w336 -> [w352 w353]
          tunnel: [w351 w353] -> w335
          tunnel: w333 -> [_ w359]
          tunnel: w332 -> [w347 w358]
          tunnel: [w347 w355] -> w331
          tunnel: w329 -> [_ w357]
          frame False {
            n147 = Increment(x=w352) -> (x+1=w351:i32)
            n148 = One Button Dialog(message="The first element of sequence was reached") -> ()  [unwired: 1 in, 1 out]
          }
          frame True {
            n149 = call "SendArrayRowToLowLevel.vi"("error in (no error)"=w358, "all rows"=w360, "Numeric"=w353, "Queue in"=w359) -> ("error out"=w356:errorcluster)  [unwired: 7 in]
            n150 = Unbundle By Name(w357) -> ("Current step"=w354:refnum<vi>)
            n151 = call "ShowCurStep.vi"("error in (no error)"=w356, "Step indicator reference"=w354, "Current step"=w353) -> ("error out"=w355:errorcluster)  [unwired: 8 in]
          }
        }
      }
      frame "NextManual" {
        n152 = Unbundle By Name(w371) -> ("SequenceQue"=w369:refnum<queue>, "LowLevelQue"=w370:refnum<queue>)
        n153 = call "IsStepLessThenSize.vi"("all rows"=w365, "Current step"=w364) -> ("Boolean"=w363:bool)  [unwired: 9 in]
        n154 = And(x=w368, y=w363) -> (x .and. y?=w367:bool)
        n155 = case shown="False" w367 {
          tunnel: w368 -> [w385 w396]
          tunnel: [w385 w396] -> w378
          tunnel: w377 -> [w384 w395]
          tunnel: [w384 w395] -> w376
          tunnel: w364 -> [w383 w394]
          tunnel: w365 -> [w382 w393]
          tunnel: [w382 w393] -> w375
          tunnel: [w383 w389] -> w374
          tunnel: w373 -> [w381 w392]
          tunnel: [w381 w388] -> w372
          tunnel: w370 -> [_ w391]
          tunnel: w369 -> [_ _]
          tunnel: w366 -> [_ w387]
          frame False {
            n156 = One Button Dialog(message="The last element of the suquence was reached") -> ()  [unwired: 1 in, 1 out]
          }
          frame True {
            n157 = Increment(x=w394) -> (x+1=w389:i32)
            n158 = call "SendArrayRowToLowLevel.vi"("error in (no error)"=w392, "all rows"=w393, "Numeric"=w389, "Queue in"=w391) -> ("error out"=w390:errorcluster)  [unwired: 7 in]
            n159 = Unbundle By Name(w387) -> ("Current step"=w386:refnum<vi>)
            n160 = call "ShowCurStep.vi"("error in (no error)"=w390, "Step indicator reference"=w386, "Current step"=w389) -> ("error out"=w388:errorcluster)  [unwired: 8 in]
          }
        }
      }
      frame "Reset" {
        w403 = -1
        n161 = Unbundle By Name(w406) -> ("Current step"=w404:refnum<vi>)
        n162 = Unbundle By Name(w398) -> ("LowLevelQue"=w397:refnum<queue>)
        n163 = call "ShowCurStep.vi"("error in (no error)"=w405, "Step indicator reference"=w404, "Current step"=w403) -> ("error out"=w402:errorcluster)  [unwired: 8 in]
        n164 = call "SendArrayRowToLowLevel.vi"("error in (no error)"=w402, "all rows"=i64[][] [], "Numeric"=0, "Queue in"=w397) -> ("error out"=w401:errorcluster)  [unwired: 7 in]
      }
      frame "Halt" {
      }
      frame "NextSequenceStep" {
        n165 = call "IsStepLessThenSize.vi"("all rows"=w419, "Current step"=w420) -> ("Boolean"=w418:bool)  [unwired: 9 in]
        n166 = And(x=w431, y=w429) -> (x .and. y?=w417:bool)
        n167 = Build Array(w418, w417) -> (w433:bool[])
        n168 = Boolean Array To Number(Boolean array=w433) -> (number=w432:u32)
        n169 = case shown="0, Default" w432 {
          tunnel: [w434 w455 w472] -> w430
          tunnel: w431 -> [w434 w455 w472]
          tunnel: w429 -> [w438 w454 w471]
          tunnel: [w438 w454 w471] -> w428
          tunnel: [w437 w441 w456] -> w427
          tunnel: w420 -> [w437 _ w464]
          tunnel: w419 -> [w436 w445 w468]
          tunnel: [w436 w445 w468] -> w426
          tunnel: w425 -> [_ w453 w470]
          tunnel: [w435 w444 w460] -> w423
          tunnel: w424 -> [w435 w440 w458]
          tunnel: w421 -> [_ w449 w465]
          frame 0, Default {
            n170 = case shown="False" w434 {
              frame False {
                n171 = One Button Dialog(message="Sequence not loaded") -> ()  [unwired: 1 in, 1 out]
              }
              frame True {
              }
            }
          }
          frame 2 {
            w441 = 0
            n172 = Unbundle By Name(w449) -> ("Current step"=w442:refnum<vi>)
            n173 = Unbundle By Name(w453) -> ("SequenceQue"=w451:refnum<queue>, "LowLevelQue"=w452:refnum<queue>)
            n174 = call "ShowCurStep.vi"("error in (no error)"=w440, "Step indicator reference"=w442, "Current step"=w441) -> ("error out"=w443:errorcluster)  [unwired: 8 in]
            n175 = call "GetTimeInSecFromArr.vi"("Current step"=w441, "all rows"=w445) -> ("Time in sec"=w447:dbl)  [unwired: 9 in]
            n176 = call "SendArrayRowToLowLevel.vi"("error in (no error)"=w443, "all rows"=w445, "Numeric"=w441, "Queue in"=w452) -> ("error out"=w448:errorcluster)  [unwired: 7 in]
            n177 = call "Time Delay"("error in (no error)"=w448, "Delay Time (s)"=w447) -> ("error out"=w446:errorcluster)  [unwired: 9 in]
            n178 = Enqueue Element(queue=w451, element=T5 {"SequenceMsg"=enum."NextSequenceStep", "Sequence String"=""}, error in (no error)=w446) -> (error out=w444:errorcluster)  [unwired: 1 in, 2 out]
          }
          frame 3 {
            n179 = Unbundle By Name(w470) -> ("SequenceQue"=w467:refnum<queue>, "LowLevelQue"=w469:refnum<queue>)
            n180 = Unbundle By Name(w465) -> ("Current step"=w457:refnum<vi>)
            n181 = Increment(x=w464) -> (x+1=w456:i32)
            n182 = call "ShowCurStep.vi"("error in (no error)"=w458, "Step indicator reference"=w457, "Current step"=w456) -> ("error out"=w459:errorcluster)  [unwired: 8 in]
            n183 = call "GetTimeInSecFromArr.vi"("Current step"=w456, "all rows"=w468) -> ("Time in sec"=w463:dbl)  [unwired: 9 in]
            n184 = call "SendArrayRowToLowLevel.vi"("error in (no error)"=w459, "all rows"=w468, "Numeric"=w456, "Queue in"=w469) -> ("error out"=w462:errorcluster)  [unwired: 7 in]
            n185 = call "Time Delay2"("error in (no error)"=w462, "Delay Time (s)"=w463) -> ("error out"=w461:errorcluster)  [unwired: 9 in]
            n186 = Enqueue Element(queue=w467, element=T5 {"SequenceMsg"=enum."NextSequenceStep", "Sequence String"=""}, error in (no error)=w461) -> (error out=w460:errorcluster)  [unwired: 1 in, 2 out]
          }
        }
      }
    }
  }
